vi "ParseVectorFile.SVG.RectFactory.vi"(8 "error in (no error)":errorcluster, 11 "ParseVectorFile in":refnum<class "ParseVectorFile.lvclass">) -> (0 "error out":errorcluster, 3 "ParseVectorFile out":refnum<class "ParseVectorFile.lvclass">)   [LabVIEW 2019, in "ParseVectorFile.lvclass"]
uses:
  ParseVectorFile.lvclass
  ParseVectorFile.lvclass/ParseVectorFile.ctl
  ParseXML/ParseSVG.lvclass/ParseSVG.ctl
  Rectangle/InitializeInformation.ctl
  Rectangle/Rectangle.lvclass
  ParseXML/ParseSVG.lvclass
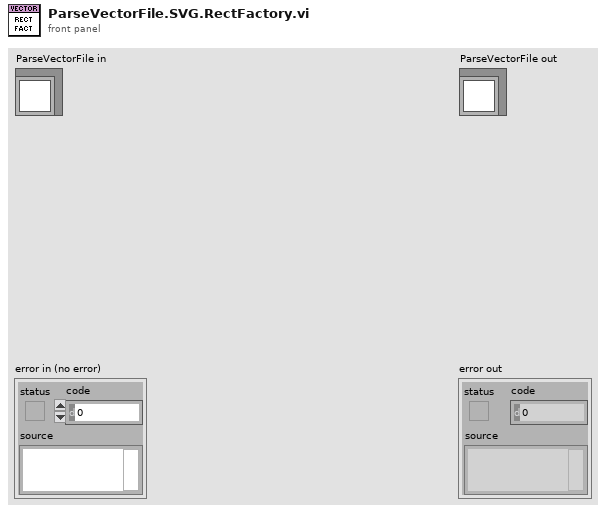
[diagram p1: front panel]
types:
  T1 = typedef "ParseSVG.lvclass/Rect.ctl" = cluster{"style":string, "transform":string, "x":string, "y":string, "width":string, "height":string, "rx":string, "ry":string, "id":string}
  T2 = typedef "Rectangle.lvclass/InitializeInformation.ctl" = cluster{"X":string, "Y":string, "Width":string, "Height":string, "Rx":string, "Ry":string}
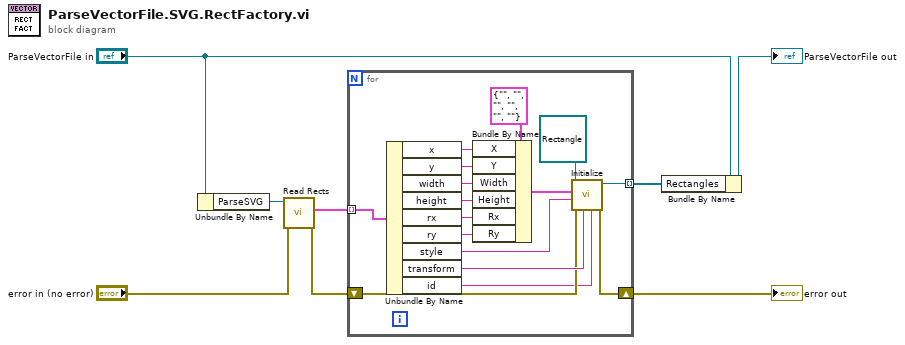
[diagram p0: block diagram]
diagram:
  n1 = Unbundle By Name("ParseVectorFile in") -> ("ParseSVG"=w6:refnum<class "ParseSVG.lvclass">)
  n2 = call "Read Rects.vi"("error in (no error)"="error in (no error)", "ParseSVG in"=w6) -> ("error out"=w7:errorcluster, "Rects"=w8:T1[])  [unwired: 7 in, 1 out]
  n3 = for {
    tunnel: w8 -> [w24] mode=indexing
    shift-right: [w11] -> w4
    shift-left: w7 -> [w12]
    tunnel: [w10] -> w1 mode=indexing
    n4 = Unbundle By Name(w24) -> ("x"=w22:string, "y"=w21:string, "width"=w20:string, "height"=w19:string, "rx"=w18:string, "ry"=w17:string, "style"=w14:string, "transform"=w13:string, "id"=w9:string)
    n5 = Bundle By Name(cluster=T2 {"X"="", "Y"="", "Width"="", "Height"="", "Rx"="", "Ry"=""} ("rect"), "X"=w22, "Y"=w21, "Width"=w20, "Height"=w19, "Rx"=w18, "Ry"=w17) -> (w15:T2)
    n6 = call "Initialize.vi"("id"=w9, "Transform"=w13, "error in (no error)"=w12, "Style"=w14, "rect"=w15, "Rectangle in"=refnum<class "Rectangle.lvclass"> refnum) -> ("error out"=w11:errorcluster, "Rectangle out"=w10:refnum<class "Rectangle.lvclass">)  [unwired: 4 in]
  }
  "error out" <- w4
  n7 = Bundle By Name(cluster="ParseVectorFile in", "Rectangles"=w1) -> (→"ParseVectorFile out":refnum<class "ParseVectorFile.lvclass">)
